vi "Store Static VI References for Subpanel.vi"(8 "error in (no error)":errorcluster, 11 "CCD Configuration in":refnum<class "CCD Configuration.lvclass">) -> (0 "error out":errorcluster, 3 "CCD Configuration out":refnum<class "CCD Configuration.lvclass">)   [LabVIEW 2016, in "CCD.lvlib" / "CCD Configuration.lvclass"]
uses:
  <userlib>/Common Components/Hardware/CCD/CCD Configuration.lvclass
  C:/Program Files (x86)/National Instruments/LabVIEW 2016/user.lib/Configuration Dialog Actor/Configuration.lvclass
  <userlib>/Configuration Dialog Actor/Configuration.lvclass
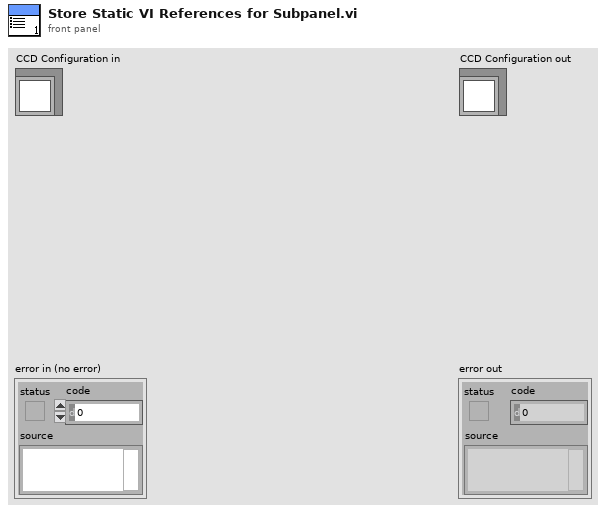
[diagram p1: front panel]
types:
  T1 = typedef "Configuration.lvlib/Configuration.lvclass/Data Retrieved by Lookup Table.ctl" = cluster{"VI Refnum":refnum<vi>, "Help Text":string}
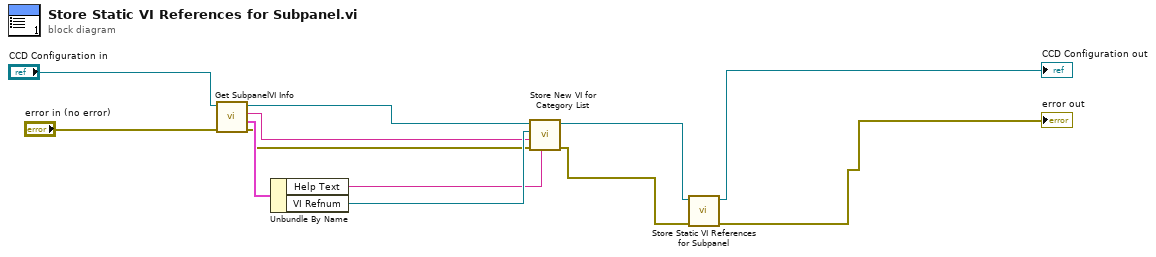
[diagram p0: block diagram]
diagram:
  n1 = call <userlib>:"Get SubpanelVI Info.vi"("error in (no error)"="error in (no error)", "Hardware.lvlib:CCD.lvlib:CCD Configuration.lvclass"="CCD Configuration in") -> ("error out"=w5:errorcluster, "Subpanel VI data"=w10:T1, "Category string"=w7:string, "reference out"=w9:refnum<class "CCD Configuration.lvclass">)  [unwired: 6 in]
  n2 = Unbundle By Name(w10) -> ("Help Text"=w6:string, "VI Refnum"=w8:refnum<vi>)
  n3 = call <userlib>:"Store New VI for Category List.vi"("Help Text"=w6, "error in (no error)"=w5, "String"=w7, "VI Refnum"=w8, "Configuration in"=w9) -> ("error out"=w3:errorcluster, "Configuration out"=w4:refnum<class "CCD Configuration.lvclass">)  [unwired: 5 in]
  n4 = call-parent "Store Static VI References for Subpanel.vi"("error in (no error)"=w3, "Configuration in"=w4) -> ("error out"=→"error out":errorcluster, "Configuration out"=→"CCD Configuration out":refnum<class "CCD Configuration.lvclass">)  [unwired: 8 in]
